vi "MatchPattern.vi"() -> ()   [LabVIEW 2019]
panel:
  out "after substring":string
  out "match substring":string
  out "before substring":string
  in  "Input String":string
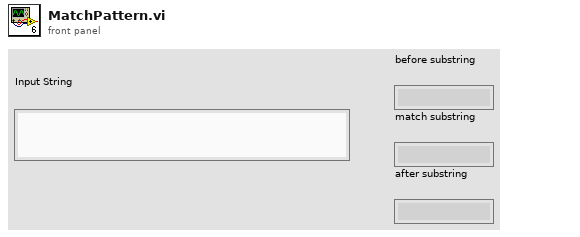
[diagram p1: front panel]
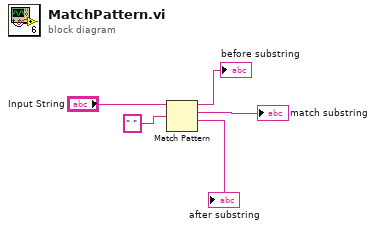
[diagram p0: block diagram]
diagram:
  n1 = Match Pattern(string="Input String", regular expression=" ") -> (before substring=→"before substring":string, match substring=→"match substring":string, after substring=→"after substring":string)  [unwired: 1 in, 1 out]
